vi "main.vi"   [LabVIEW 2015]
uses:
  SYS/Master Controller_llb/Master Controller.lvclass
types:
  T1 = enum32{"invalid app kind", "Development System", "Run Time System", "Student Edition", "Embedded LabVIEW", "Evaluation", "Custom"}
  T2 = enum32{"Invalid", "Standard", "Closed", "Hidden", "Minimized", "Maximized"}
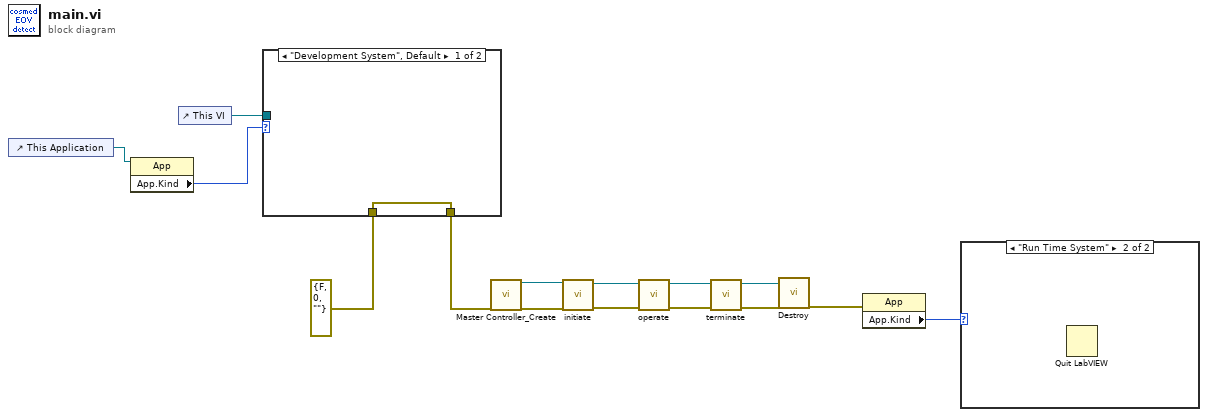
[diagram p0: block diagram]
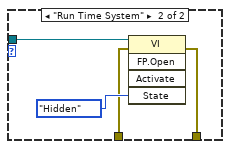
[diagram p3: hidden frame]
diagram:
  n1 = control-ref of="This Application"() -> (w4:refnum<vi>)
  n2 = property class="App"(reference=w4) -> ("App.Kind"=w3:T1)  [unwired: 1 in, 2 out]
  n3 = control-ref of="This VI"() -> (w5:refnum<vi>)
  n4 = case shown="\"Development System\", Default" w3 {
    tunnel: w5 -> [_ w20]
    tunnel: errorcluster {"status"=FALSE, "code"=0, "source"=""} ("error in (no error)") -> [w16 w18]
    tunnel: [w16 w17] -> w6
    frame "Development System", Default {
    }
    frame "Run Time System" {
      n5 = invoke class="VI" method="FP.Open"(reference=w20, error in=w18, "State"=T2."Hidden") -> (error out=w17:errorcluster)  [unwired: 2 in, 4 out]
    }
  }
  n6 = call "Master Controller_Create.vi"("error in (no error)"=w6) -> ("reference out"=w14:refnum<class "Master Controller.lvclass">, "error out"=w15:errorcluster)  [unwired: 17 in]
  n7 = call "initiate.vi"("error in (no error)"=w15, "reference in"=w14) -> ("error out"=w13:errorcluster, "reference out"=w12:refnum<class "Master Controller.lvclass">)  [unwired: 8 in]
  n8 = call "operate.vi"("error in (no error)"=w13, "reference in"=w12) -> ("error out"=w11:errorcluster, "reference out"=w10:refnum<class "Master Controller.lvclass">)  [unwired: 8 in]
  n9 = call "terminate.vi"("error in (no error)"=w11, "reference in"=w10) -> ("error out"=w9:errorcluster, "reference out"=w8:refnum<class "Master Controller.lvclass">)  [unwired: 8 in]
  n10 = call-dynamic "Destroy.vi"("reference in"=w8, "error in (no error)"=w9) -> ("error out"=w2:errorcluster)  [unwired: 16 in, 1 out]
  n11 = property class="App"(error in=w2) -> ("App.Kind"=w1:T1)  [unwired: 1 in, 2 out]
  n12 = case shown="\"Run Time System\"" w1 {
    frame "Development System", Default {
    }
    frame "Run Time System" {
      n13 = Quit LabVIEW() -> ()  [unwired: 1 in]
    }
  }
